vi "Stop Core.vi"(10 "final error code":i32, 11 "Guardian in":refnum<class "Guardian.lvclass">) -> (3 "Guardian out":refnum<class "Guardian.lvclass">)   [LabVIEW 2026, in "TALOS.lvlib" / "Guardian.lvlib" / "Guardian.lvclass"]
doc: "(<B>Filename</B>: Actor Framework.lvlib:Actor.lvclass:Stop Core.vi)\n\nDefines what the actor does before it stops. Use the <B>final error code</B> input to determine whether the actor shut down in response to an error.\n\nBy default, this method passes the Stop message along to all auto-stop nested actors. A descendant class may override this method to define additional behavior, such as shutting down any processes the actor initiated in its override of the Actor Core method."
uses:
  Guardian.lvclass
  Ancestor/Ancestor/Ancestor.lvclass
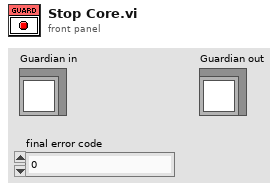
[diagram p1: front panel]
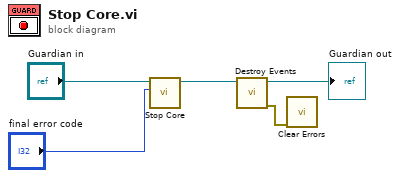
[diagram p0: block diagram]
diagram:
  n1 = call-parent "Stop Core.vi"("final error code"="final error code", "Ancestor in"="Guardian in") -> ("Ancestor out"=w4:refnum<class "Guardian.lvclass">)  [unwired: 9 in]
  n2 = call-dynamic "Destroy Events.vi"("Guardian in"=w4) -> ("error out"=w1:errorcluster, "Guardian out"=→"Guardian out":refnum<class "Guardian.lvclass">)  [unwired: 9 in]
  n3 = call <vilib>:"Clear Errors.vi"("error in (no error)"=w1) -> ()  [unwired: 5 in, 2 out]
